vi "Set Data Depth.vi"(0 "New Buffer Size":i32, 1 "Plugin Names":T2, 3 "error in (no error)":errorcluster) -> (4 "Result":T1=enum."Update Failed", 5 "New Buffer Size out":i32, 6 "Plugin Names out":T2, 7 "Changed?":bool, 8 "error out":errorcluster)   [LabVIEW 2015, in "Config Data.lvlib" / "Config Data.lvclass"]
uses:
  Config Data.lvclass
  Startup Processes/_typedefs/Subpanel Names.ctl
  Startup Processes/_typedefs/Pass Fail Flag.ctl
  Startup Processes/Startup Processes.lvlib
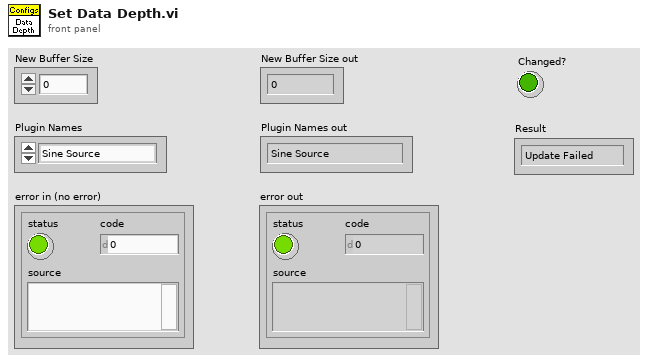
[diagram p1: front panel]
types:
  T1 = typedef "Startup Processes.lvlib/Pass Fail Flag.ctl" = enum16{"Update Good", "Update Failed"}
  T2 = typedef "Startup Processes.lvlib/Subpanel Names.ctl" = enum16{"Sine Source", "Ramp Source", "Hen House TC", "Dog House TC", "Out House TC"}
  T3 = typedef "Startup Processes.lvlib/Data Valid Flag.ctl" = enum16{"Data Valid", "Data Not Valid"}
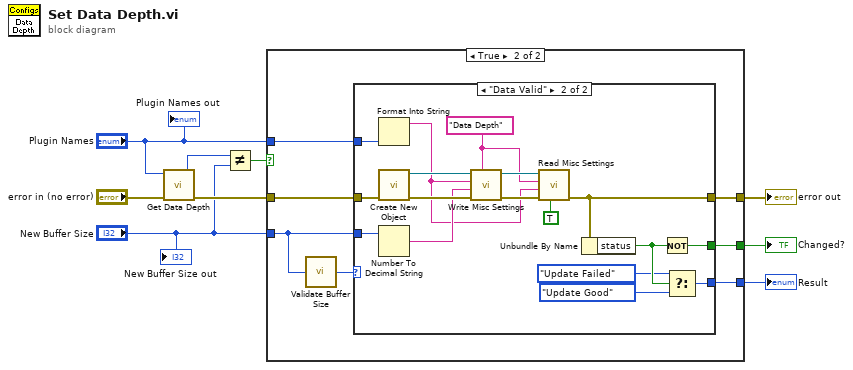
[diagram p0: block diagram]
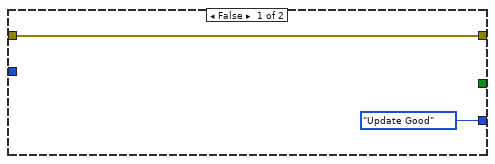
[diagram p2: hidden frame]
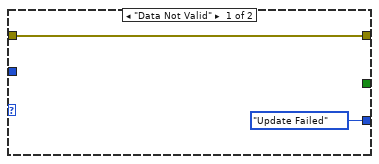
[diagram p3: hidden frame]
diagram:
  n1 = call "Get Data Depth.vi"("error in (no error)"="error in (no error)", "Depth to fetch"="Plugin Names") -> ("error out"=w7:errorcluster, "Data Depth"=w5:i32)  [unwired: 4 in]
  n2 = Not Equal?(x=w5, y="New Buffer Size") -> (x != y?=w6:bool)
  n3 = case shown="True" w6 {
    tunnel: "New Buffer Size" -> [_ w13]
    tunnel: [w11 w16] -> w9
    tunnel: w7 -> [w11 w18]
    tunnel: "Plugin Names" -> [_ w17]
    tunnel: [_ w15] -> w2
    tunnel: [Pass_Fail_Flag."Update Good" ("f") w14] -> w1
    frame False {
    }
    frame True {
      n4 = call "Validate Buffer Size.vi"("New Buffer Size"=w13) -> ("Result"=w12:T3)
      n5 = case shown="\"Data Valid\"" w12 {
        tunnel: w13 -> [_ w37]
        tunnel: w18 -> [w20 w33]
        tunnel: w17 -> [_ w32]
        tunnel: [w20 w24] -> w16
        tunnel: [_ w31] -> w15
        tunnel: [Pass_Fail_Flag."Update Failed" ("f") w29] -> w14
        frame "Data Not Valid" {
        }
        frame "Data Valid" {
          w22 = "Data Depth" ("format string")
          n6 = Format Into String(w32) -> (resulting string=w21:string)  [unwired: 3 in, 1 out]
          n7 = call "Create New Object.vi"("Error In"=w33) -> ("Error Out"=w36:errorcluster, "Config Data"=w35:refnum<class "Config Data.lvclass">)  [unwired: 5 in]
          n8 = Number To Decimal String(number=w37) -> (decimal integer string=w34:string)  [unwired: 1 in]
          n9 = call-dynamic "Write Misc Settings.vi"("Section"=w22, "error in (no error)"=w36, "p_value"=w34, "Key"=w21, "Config Data in"=w35) -> ("error out"=w25:errorcluster, "Config Data out"=w26:refnum<class "Config Data.lvclass">)  [unwired: 2 in]
          n10 = call-dynamic "Read Misc Settings.vi"("Reload"=TRUE, "error in (no error)"=w25, "Key"=w21, "Section"=w22, "Config Data in"=w26) -> ("error out"=w24:errorcluster)  [unwired: 1 in, 2 out]
          n11 = Unbundle By Name(w24) -> ("status"=w30:bool)
          n12 = Not(x=w30) -> (.not. x?=w31:bool)
          n13 = Select(t=Pass_Fail_Flag."Update Failed" ("Result"), s=w30, f=Pass_Fail_Flag."Update Good") -> (s? t:f=w29:T1)
        }
      }
    }
  }
  "error out" <- w9
  "Changed?" <- w2
  "Result" <- w1
  "New Buffer Size out" <- "New Buffer Size"
  "Plugin Names out" <- "Plugin Names"
